vi "main_ctrl.vi"(8 "error in":errorcluster) -> (0 "error out":errorcluster caption="Error")   [LabVIEW 2013]
uses:
  <vilib>/Rock Robotics/WPI/DriverStation/WPI_DriverStationRobotMode2.ctl
  typedefs/Test/test data.ctl
  typedefs/Test/test controls.ctl
  typedefs/fg_typedef.ctl
  typedefs/Vision/vision enable.ctl
  typedefs/State Machine/subStates.ctl
  typedefs/State Machine/singleUseSubstate.ctl
  <vilib>/Rock Robotics/WPI/Solenoid/WPI_SolenoidValue.ctl
  <vilib>/Rock Robotics/WPI/Compressor/WPI_CompressorGetSetRefNum.vi
  <vilib>/Rock Robotics/WPI/RobotDrive/WPI_RobotDriveGetSetRefNum.vi
  <vilib>/Rock Robotics/WPI/RobotDrive/WPI_RobotDriveArcadeDrive_Standard(NoSaturation).vi
  <vilib>/Rock Robotics/WPI/Solenoid/WPI_SolenoidSetEnum.vi
  state machine master/Cancel State Machine - Pickup.vi
  state machine master/Cancel State Machine - Load.vi
  typedefs/Vision/vision data.ctl
panel:
  out "vision errors":errorcluster
  in  "Test\nControls":T1 {"Belts" scale=-1.0..1.0; "Arm" scale=-1.0..1.0; "Drive Train" scale=-1.0..1.0}
  out "Test Data":T2
  out "Robot Mode":T3
  out "Vision mSPI":u32
  out "Vision IPS":dbl
  out "Main IPS":dbl
  out "Main mSPI":u32
  # "Test Input/Output"
  # "MAIN CONTROL"
  # "holds robot control code - dual parallel state machine"
  # "SPI: milliseconds per iteration\nIPS: iterations per second"
  # "Pneumatics"
  # "Home Encoders"
  # "Manual Override"
  # "Joystick Control"
  # "Arm Safeties"
  # "Sensors"
  # "Drive Encoders"
  # "Pneumatics Commands"
  # "Arm Encoder"
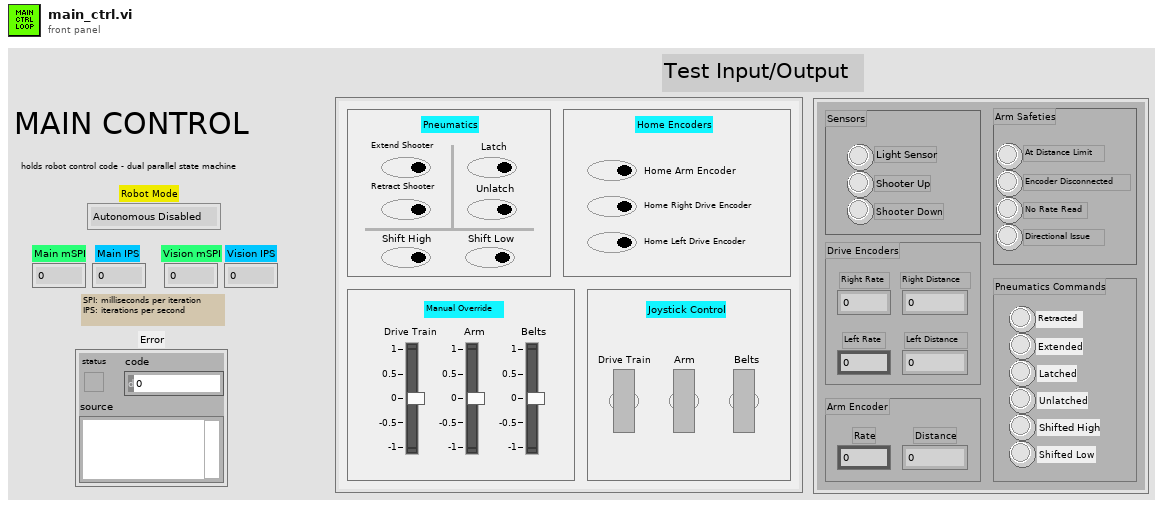
[diagram p1: front panel]
types:
  T1 = typedef "test controls.ctl" = cluster{"Drive Train":dbl, "Arm":dbl, "Belts":dbl, "Drive Train":bool, "Arm":bool, "Belts":bool, "Home Arm Encoder":bool, "Home Right Drive Encoder":bool, "Home Left Drive Encoder":bool, "Extend Shooter":bool, "Retract Shooter":bool, "Latch":bool, "Unlatch":bool, "Shift High":bool, "Shift Low":bool}
  T2 = typedef "test data.ctl" = cluster{"Light Sensor":bool, "Shooter Up":bool, "Shooter Down":bool, "Left Rate":dbl, "Left Distance":dbl, "Right Rate":dbl, "Right Distance":dbl, "Rate":dbl, "Distance":dbl, "At Distance Limit":bool, "Encoder Disconnected":bool, "No Rate Read":bool, "Directional Issue":bool, "Latched":bool, "Unlatched":bool, "Shifted High":bool, "Shifted Low":bool, "Extended":bool, "Retracted":bool}
  T3 = typedef "WPI_DriverStationRobotMode2.ctl" = enum16{"Autonomous Disabled", "Autonomous Enabled", "Teleop Disabled", "Teleop Enabled", "Timeout", "Finish", "Test Disabled", "Test Enabled"}
  T4 = typedef "fg_typedef.ctl" = enum16{"Get", "Set"}
  T5 = typedef "vision data.ctl" = cluster{"x":dbl, "y":dbl, "area":dbl, "width":dbl, "height":dbl, "Hot Goal Present?":bool, "distance":dbl}
  T6 = typedef "vision enable.ctl" = enum16{"Enable", "Disable", "Stop"}
  T7 = typedef "WPI_CameraDevRef.ctl" = cluster{"Camera Address":string, "CameraStatus":errorcluster, "Acquire Image Notifier":refnum<notifier>}
  T8 = typedef "IMAQ Image.ctl" = refnum<image>
  T9 = cluster{"Vision mSPI":u32, "Main mSPI":u32, "Dash mSPI":u32}
  T10 = typedef "WPI_RobotDriveDevRef.ctl" = cluster{"DevStatus":errorcluster, "Motors[]":T11[], "Square Inputs":bool, "Max Output":dbl, "Isochronous":bool}
  T11 = typedef "WPI_MotorControlDeviceRef.ctl" = cluster{"DeviceStatus":errorcluster, "Type":enum16{"PWM", "CAN"}, "PWM":cluster{"Digital Module":T12, "PWM Channel":T13, "DeadBand":T14}, "CAN":cluster{"Device Number":u8, "Control Mode":T15, "Semaphore":T16, "Max Vout":dbl}, "Invert":bool, "TransformRef":T17, "InvTransformRef":T17}
  T12 = typedef "FPGA_TypedefDigitalModule.ctl" = enum16{"Digital Module 1", "Digital Module 2"}
  T13 = typedef "FPGA_DIOPWMChannel.ctl" = enum8{"PWM 1", "PWM 2", "PWM 3", "PWM 4", "PWM 5", "PWM 6", "PWM 7", "PWM 8", "PWM 9", "PWM 10", "Invalid"}
  T14 = typedef "WPI_PWMDeadband.ctl" = cluster{"Name":string, "maxPositivePwm":i32, "minPositivePwm":i32, "centerPwm":i32, "maxNegativePwm":i32, "minNegativePwm":i32, "angularRange":u16}
  T15 = typedef "WPI_CANJaguar_ControlMode.ctl" = enum8{"Percent VBus", "Current", "Speed", "Position", "Voltage"}
  T16 = typedef "Semaphore RefNum" = refnum<k1>
  T17 = typedef "WPI_PWMTransform_ConPane.ctl" = refnum<vi>
  T18 = typedef "WPI_SolenoidDevRef.ctl" = cluster{"DevStatus":errorcluster, "Solenoid Module":T19, "Forward Solenoid Channel":T20, "Reverse Solenoid Channel":T20}
  T19 = typedef "FPGA_TypedefSolenoidModule.ctl" = enum16{"Solenoid Module 1", "Solenoid Module 2"}
  T20 = typedef "WPI_SolenoidChannel.ctl" = enum8{"Solenoid 1", "Solenoid 2", "Solenoid 3", "Solenoid 4", "Solenoid 5", "Solenoid 6", "Solenoid 7", "Solenoid 8", "Invalid"}
  T21 = typedef "WPI_CompressorDevRef.ctl" = cluster{"DevStatus":errorcluster, "DigitalInputDevRef":T22, "RelayDevRef":T24}
  T22 = typedef "WPI_DigitalInputDevRef.ctl" = cluster{"DevStatus":errorcluster, "DIO Channel":T23, "Digital Module":T12}
  T23 = typedef "FPGA_DIOChannel.ctl" = enum8{"DIO 1", "DIO 2", "DIO 3", "DIO 4", "DIO 5", "DIO 6", "DIO 7", "DIO 8", "DIO 9", "DIO 10", "DIO 11", "DIO 12", "DIO 13", "DIO 14", "Invalid"}
  T24 = typedef "WPI_RelayDevRef.ctl" = cluster{"DevStatus":errorcluster, "Relay Channel":T25, "Digital Module":T12, "Relay Direction":T26}
  T25 = typedef "FPGA_DIORelayChannel.ctl" = enum8{"Relay 1", "Relay 2", "Relay 3", "Relay 4", "Relay 5", "Relay 6", "Relay 7", "Relay 8", "Invalid"}
  T26 = typedef "WPI_RelayDirection.ctl" = enum16{"Both directions", "Forward only", "Reverse only"}
  T27 = typedef "WPI_SolenoidValue.ctl" = enum16{"Off", "On", "Forward", "Reverse"}
  T28 = typedef "subStates.ctl" = enum16{"null", "wait", "driver control", "auto", "manual override", "hold position", "rotate", "pickup", "pass", "recover pass", "load", "goto shoot", "shoot high goal", "shoot low goal", "cancel arm", "cancel shooter", "end", "test"}
  T29 = typedef "singleUseSubstate.ctl" = enum16{"null", "wait", "shift high", "shift low", "extend shooter", "retract shooter", "latch", "unlatch", "end"}
  T30 = typedef "WPI_DriverStationDerivedRobotMode.ctl" = enum16{"Init", "Execute", "Stop"}
  T31 = typedef "Loop 2 Datatype.ctl" = cluster{"State":T28, "Waiting Loop":i32, "State to Wait For":i32, "Loop ID":i32, "Exit Value":i32, "Joystick Y":dbl, "Joystick Z":dbl}
  T32 = typedef "Loop 1 Datatype.ctl" = cluster{"State":T28, "Waiting Loop":i32, "State to Wait For":i32, "Loop ID":i32, "Exit Value":i32}
  T33 = typedef "Loop 3 Datatype.ctl" = cluster{"State":T28, "Waiting Loop":i32, "State to Wait For":i32, "Loop ID":i32, "Exit Value":i32, "Joystick Y":dbl, "Tune Setpoint":cluster{"Increment":bool, "Decrement":bool}}
  T34 = typedef "Loop 0 Datatype.ctl" = cluster{"State":T28, "Waiting Loop":i32, "State to Wait For":i32, "Loop ID":i32, "Exit Value":i32, "X Axis":dbl, "Y Axis":dbl, "Z Axis":dbl}
  T35 = typedef "dashboard safety status data.ctl" = cluster{"At Distance Limit":bool, "No Rate Read":bool, "Encoder Disconnected":bool, "Encoder Directional Issue":bool}
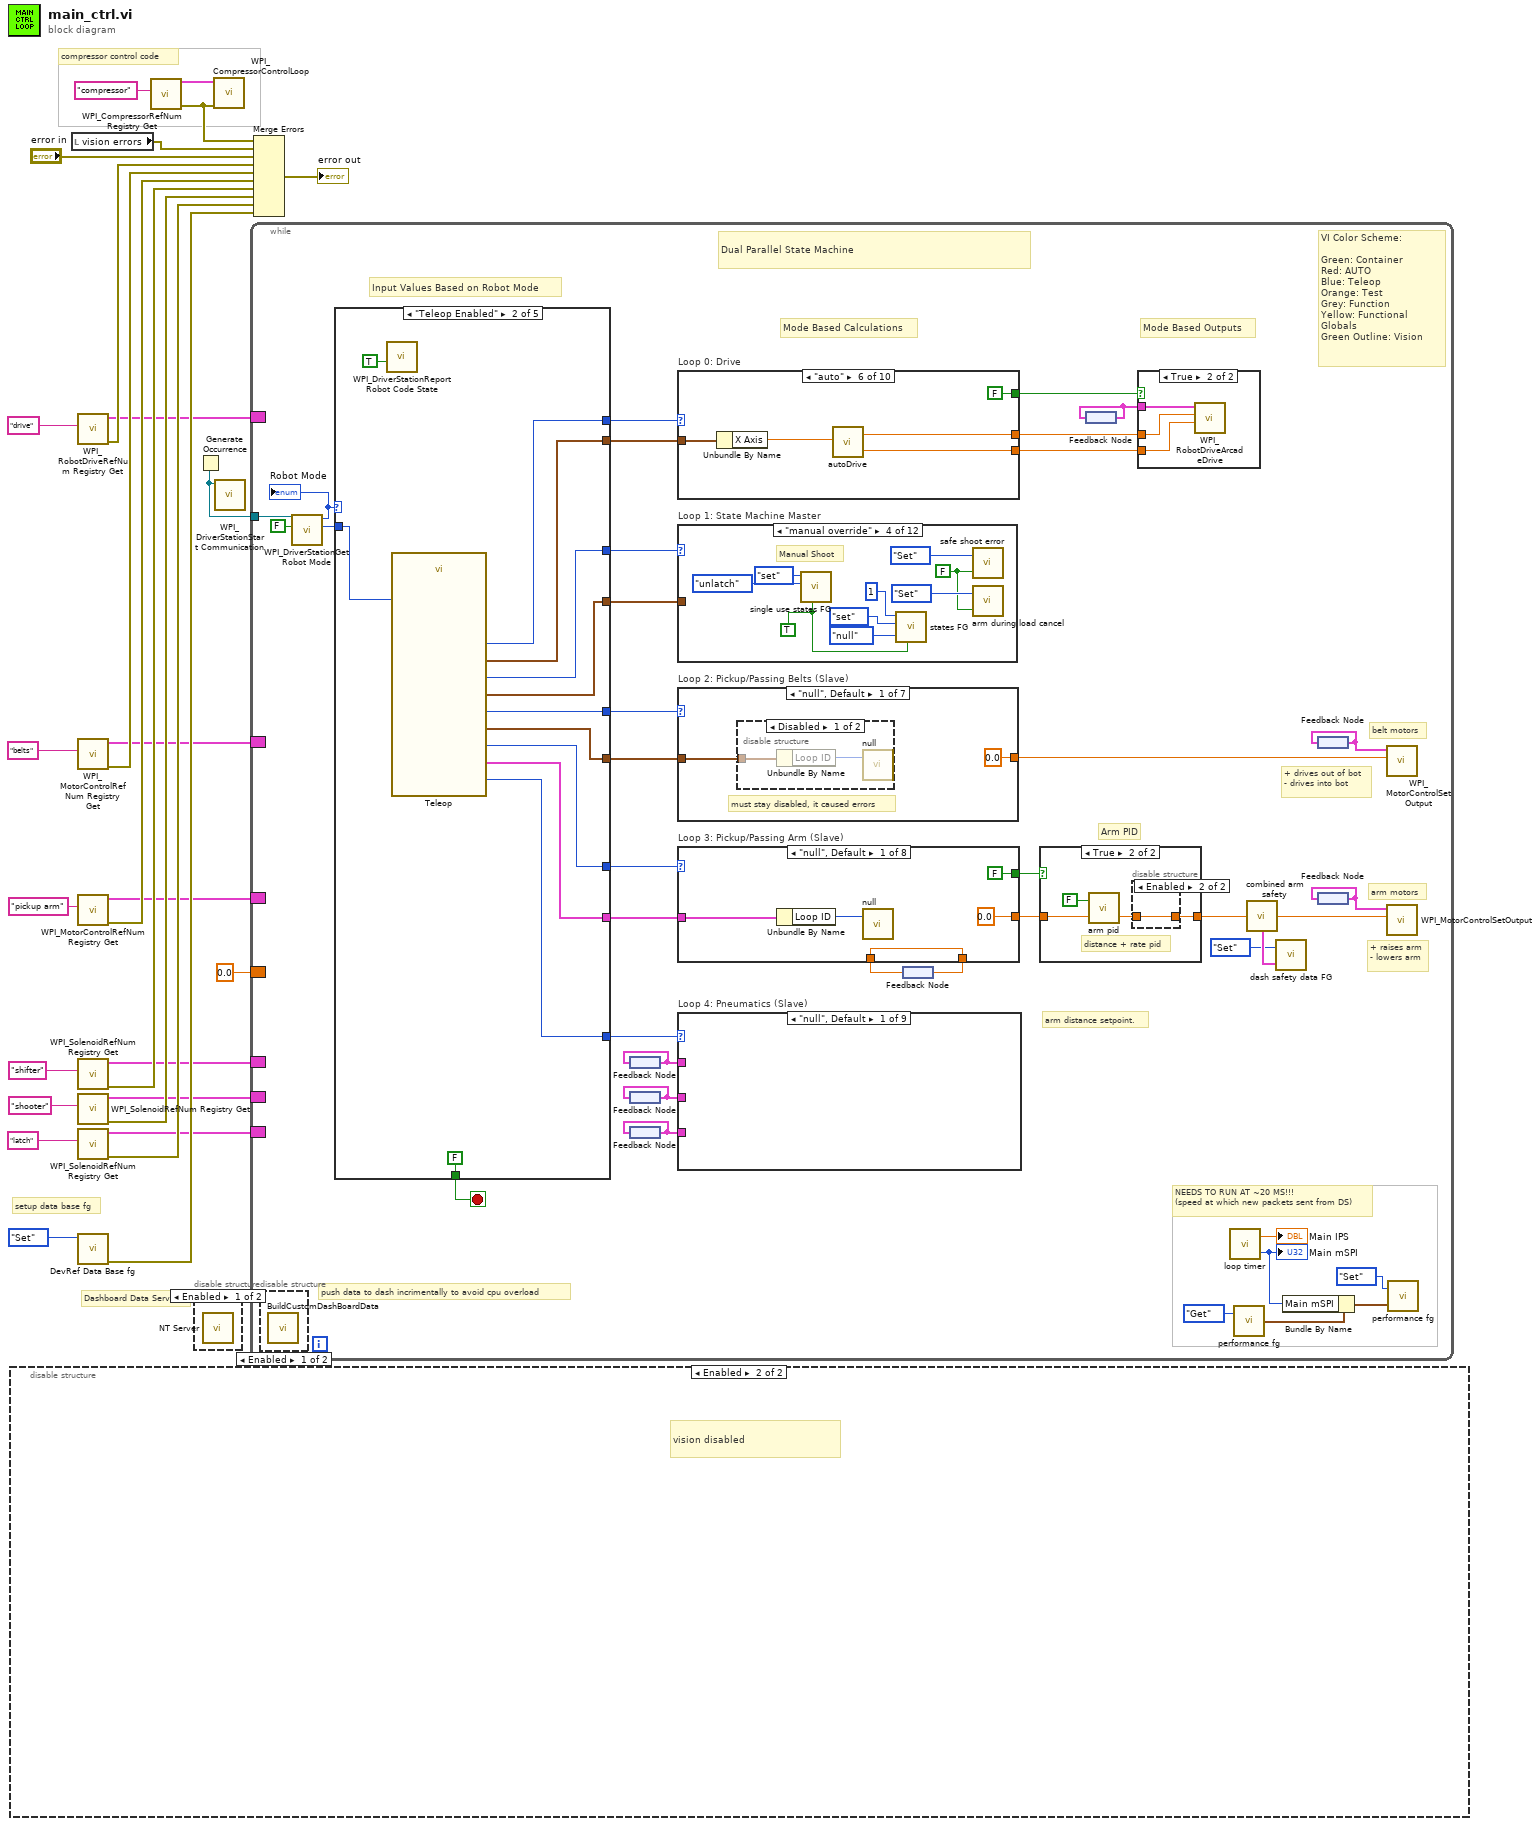
[diagram p0: block diagram]
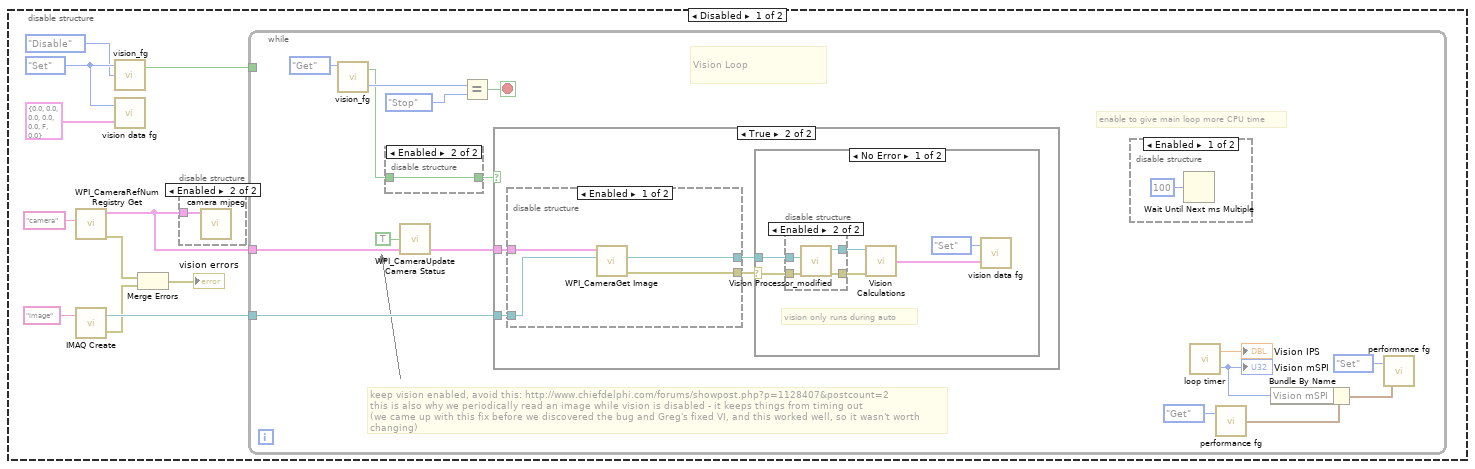
[diagram p3: hidden frame]
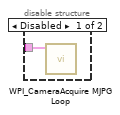
[diagram p4: hidden frame]
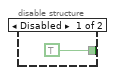
[diagram p5: hidden frame]
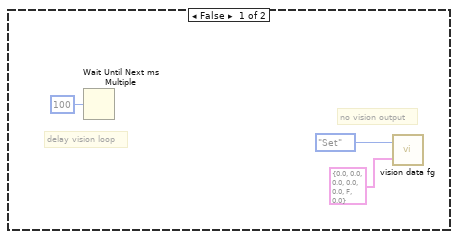
[diagram p7: hidden frame]
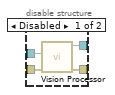
[diagram p8: hidden frame]
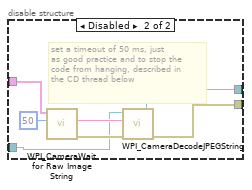
[diagram p10: hidden frame]
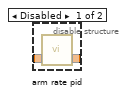
[diagram p12: hidden frame]
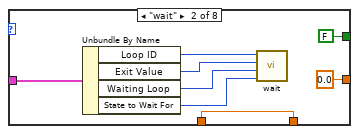
[diagram p13: hidden frame]
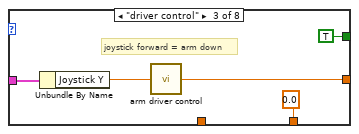
[diagram p14: hidden frame]
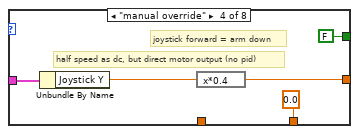
[diagram p15: hidden frame]
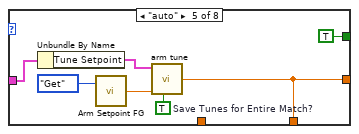
[diagram p16: hidden frame]
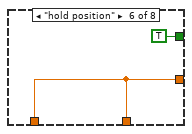
[diagram p17: hidden frame]
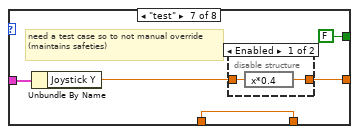
[diagram p18: hidden frame]
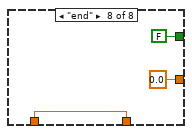
[diagram p20: hidden frame]
diagram:
  # "compressor control code"
  # "Dashboard Data Server"
  # "setup data base fg"
  n1 = disable-structure shown="Enabled" {
    frame Disabled {
      w37 = fg_typedef."Set" ("Enum")
      n2 = call <vilib>:"WPI_CameraRefNum Registry Get.vi"("refnum name"="camera") -> ("error out"=w30:errorcluster, "CameraDevRef"=w34:T7)  [unwired: 9 in]
      n3 = call "IMAQ Create"("Image Name"="image") -> ("New Image"=w39:T8, "error out"=w31:errorcluster)  [unwired: 4 in]
      n4 = call "vision_fg.vi"("Action"=vision_enable."Disable", "Menu"=w37) -> ("Enabled?"=w38:bool)  [unwired: 1 in, 1 out]
      n5 = call "vision data fg.vi"("Input"=T5 {"x"=0.0, "y"=0.0, "area"=0.0, "width"=0.0, "height"=0.0, "Hot Goal Present?"=FALSE, "distance"=0.0} ("Cluster"), "Menu"=w37) -> ()  [unwired: 1 out]
      n6 = Merge Errors(w30, w31) -> (→"vision errors":errorcluster)
      n7 = disable-structure shown="Enabled" {
        disable-tunnel: w34 -> [w40 w41]
        frame Disabled {
          n8 = call <vilib>:"WPI_CameraAcquire MJPG Loop.vi"("CameraDevRef"=w40) -> ()  [unwired: 11 in]
        }
        frame Enabled {
          n9 = call "camera mjpeg.vi"("CameraDevRef"=w41) -> ()  [unwired: 11 in]
        }
      }
      n10 = while {
        tunnel: w39 -> [w56]
        tunnel: w34 -> [w55]
        tunnel: w38 -> [_]
        stop <- w57 stop-if-true
        # "keep vision enabled, avoid this: http://www.chiefdelphi.com/forums/showpost.php?p=1128407&postcount=2\nthis is also why we periodically read an image while vision is disabled - it keeps things from timing out\n(we came up with this fix before we discovered the bug and Greg's fixed VI, and this worked well, so it wasn't worth changing)"
        # "enable to give main loop more CPU time"
        # "Vision Loop"
        n11 = call "vision_fg.vi"("Menu"=fg_typedef."Get" ("Enum")) -> ("State Out"=w51:T6, "Enabled?"=w42:bool)  [unwired: 2 in]
        n12 = disable-structure shown="Enabled" {
          disable-tunnel: [TRUE w59] -> w43
          disable-tunnel: w42 -> [_ w59]
          frame Disabled {
          }
          frame Enabled {
          }
        }
        n13 = call <vilib>:"WPI_CameraUpdate Camera Status.vi"("CameraDevRef In"=w55, "Enable Vision"=TRUE) -> ("CameraDevRef Out"=w54:T7)  [unwired: 3 in]
        n14 = Equal?(x=w51, y=vision_enable."Stop") -> (x = y?=w57:bool)
        n15 = case shown="True" w43 {
          tunnel: w56 -> [_ w67]
          tunnel: w54 -> [_ w66]
          frame False {
            # "no vision output"
            # "delay vision loop"
            n16 = Wait Until Next ms Multiple(millisecond multiple=u32 100) -> ()  [unwired: 1 out]
            n17 = call "vision data fg.vi"("Input"=T5 {"x"=0.0, "y"=0.0, "area"=0.0, "width"=0.0, "height"=0.0, "Hot Goal Present?"=FALSE, "distance"=0.0} ("Cluster"), "Menu"=fg_typedef."Set" ("Enum")) -> ()  [unwired: 1 out]
          }
          frame True {
            n18 = disable-structure shown="Enabled" {
              disable-tunnel: w67 -> [w84 w88]
              disable-tunnel: w66 -> [w85 w90]
              disable-tunnel: [w83 w87] -> w65
              disable-tunnel: [w82 w86] -> w64
              frame Enabled {
                n19 = call <vilib>:"WPI_CameraGet Image.vi"("Image"=w84, "CameraDevRef"=w85) -> ("error out"=w82:errorcluster, "Image Out"=w83:T8)  [unwired: 7 in, 1 out]
              }
              frame Disabled {
                # "set a timeout of 50 ms, just\nas good practice and to stop the \ncode from hanging, described in \nthe CD thread below"
                n20 = call <vilib>:"WPI_CameraWait for Raw Image String.vi"("Timeout in ms (-1)"=50, "CameraDevRef"=w90) -> ("error out"=w92:errorcluster, "String"=w91:string)  [unwired: 3 in, 5 out]
                n21 = call <vilib>:"WPI_CameraDecodeJPEGString.vi"("error in"=w92, "Compressed Image"=w91, "Image In"=w88) -> ("error out"=w86:errorcluster, "Image Out"=w87:T8)  [unwired: 3 out]
              }
            }
            n22 = case shown="No Error" w64 {
              selector: w64 -> [w72 _]
              tunnel: w65 -> [w71 _]
              frame No Error {
                # "vision only runs during auto"
                n23 = disable-structure shown="Enabled" {
                  disable-tunnel: w72 -> [w77 w80]
                  disable-tunnel: w71 -> [w76 w81]
                  disable-tunnel: [w75 w78] -> w70
                  disable-tunnel: [w74 w79] -> w69
                  frame Disabled {
                    n24 = call "Vision Processor.vi"("error in"=w77, "Image In"=w76) -> ("error out"=w74:errorcluster, "Image Out"=w75:T8)  [unwired: 5 in]
                  }
                  frame Enabled {
                    n25 = call "Vision Processor_modified.vi"("error in"=w80, "Image In"=w81) -> ("error out"=w79:errorcluster, "Image Out"=w78:T8)  [unwired: 5 in]
                  }
                }
                n26 = call "Vision Calculations.vi"("Image In"=w70, "error in"=w69) -> ("Vision Data"=w68:T5)  [unwired: 3 in]
                n27 = call "vision data fg.vi"("Input"=w68, "Menu"=fg_typedef."Set" ("Enum")) -> ()  [unwired: 1 out]
              }
              frame Error {
              }
            }
          }
        }
        n28 = disable-structure shown="Enabled" {
          frame Enabled {
            n29 = Wait Until Next ms Multiple(millisecond multiple=u32 100) -> ()  [unwired: 1 out]
          }
          frame Disabled {
          }
        }
        n30 = call "loop timer.vi"() -> ("IPS"=→"Vision IPS":dbl, "SPI"=w49:u32)  [unwired: 1 in]
        "Vision mSPI" <- w49
        n31 = call "performance fg.vi"("Menu"=fg_typedef."Get") -> ("Output"=w47:T9)  [unwired: 1 in]
        n32 = Bundle By Name(cluster=w47, "Vision mSPI"=w49) -> (w46:T9)
        n33 = call "performance fg.vi"("Input"=w46, "Menu"=fg_typedef."Set") -> ()  [unwired: 1 out]
      }
    }
    frame Enabled {
      # "vision disabled"
    }
  }
  n34 = local read "vision errors"() -> (w1:errorcluster)
  n35 = call <vilib>:"WPI_RobotDriveRefNum Registry Get.vi"("refnum name"="drive") -> ("error out"=w27:errorcluster, "RobotDriveDevRef"=w3:T10)  [unwired: 9 in]
  n36 = call <vilib>:"WPI_MotorControlRefNum Registry Get.vi"("refnum name"="belts") -> ("error out"=w26:errorcluster, "MotorControlDevRef"=w7:T11)  [unwired: 9 in]
  n37 = call <vilib>:"WPI_MotorControlRefNum Registry Get.vi"("refnum name"="pickup arm") -> ("error out"=w25:errorcluster, "MotorControlDevRef"=w10:T11)  [unwired: 9 in]
  n38 = call <vilib>:"WPI_SolenoidRefNum Registry Get.vi"("refnum name"="shifter") -> ("error out"=w24:errorcluster, "SolenoidDevRef"=w17:T18)  [unwired: 9 in]
  n39 = call <vilib>:"WPI_SolenoidRefNum Registry Get.vi"("refnum name"="shooter") -> ("error out"=w23:errorcluster, "SolenoidDevRef"=w5:T18)  [unwired: 9 in]
  n40 = call <vilib>:"WPI_SolenoidRefNum Registry Get.vi"("refnum name"="latch") -> ("error out"=w22:errorcluster, "SolenoidDevRef"=w6:T18)  [unwired: 9 in]
  n41 = call "DevRef Data Base fg.vi"("Menu"=fg_typedef."Set") -> ("error out"=w28:errorcluster)  [unwired: 3 in, 5 out]
  n42 = call <vilib>:"WPI_CompressorRefNum Registry Get.vi"("refnum name"="compressor") -> ("error out"=w2:errorcluster, "CompressorDevRef"=w18:T21)  [unwired: 9 in]
  n43 = disable-structure shown="Enabled" {
    frame Enabled {
      n44 = call <vilib>:"NT Server.vi"() -> ()  [unwired: 12 in]
    }
    frame Disabled {
    }
  }
  n45 = Generate Occurrence() -> (w15:refnum<k4>)
  n46 = call <vilib>:"WPI_CompressorControlLoop.vi"("error in (no error)"=w2, "CompressorDevRef"=w18) -> ()  [unwired: 10 in]
  n47 = call <vilib>:"WPI_DriverStationStart Communication.vi"("occurrence"=w15) -> ()  [unwired: 11 in]
  n48 = while {
    tunnel: w15 -> [w110]
    border: w3 -> [_]
    border: w17 -> [_]
    border: w6 -> [_]
    border: w5 -> [_]
    border: w7 -> [_]
    border: w10 -> [_]
    border: 0.0 ("setpoint") -> [_]
    stop <- w127 stop-if-true
    # "Arm PID"
    # "Mode Based Outputs"
    # "arm motors"
    # "arm distance setpoint."
    # "push data to dash incrimentally to avoid cpu overload"
    # "+ raises arm\n- lowers arm"
    # "+ drives out of bot\n- drives into bot"
    # "belt motors"
    # "VI Color Scheme:\n\nGreen: Container\nRed: AUTO\nBlue: Teleop\nOrange: Test \nGrey: Function\nYellow: Functional Globals\nGreen Outline: Vision"
    # "Input Values Based on Robot Mode"
    # "Mode Based Calculations"
    # "NEEDS TO RUN AT ~20 MS!!!\n(speed at which new packets sent from DS)"
    # "Dual Parallel State Machine"
    n49 = disable-structure shown="Enabled" {
      frame Enabled {
        n50 = call "BuildCustomDashBoardData.vi"() -> ()  [unwired: 12 in]
      }
      frame Disabled {
      }
    }
    n51 = call <vilib>:"WPI_DriverStationGet Robot Mode.vi"("Finish"=FALSE, "DS Occurrence"=w110) -> ("Call Context"=w109:T30, "Robot Mode"=w108:T3)  [unwired: 8 out]
    "Robot Mode" <- w108
    n52 = case shown="\"Teleop Enabled\"" w108 {
      tunnel: [w316 w331 w340 w348 w354] -> w112
      tunnel: w109 -> [w309 w327 w343 _ _]
      tunnel: [w314 w330 w342 w348 w354] -> w129
      tunnel: [w310 w328 w334 singleUseSubstate."null" ("SubState 5") singleUseSubstate."end" ("SubState 5")] -> w128
      tunnel: [FALSE FALSE FALSE FALSE TRUE] -> w127
      tunnel: [w318 w326 w338 w348 w354] -> w102
      tunnel: [w317 w325 w339 _ _] -> w121
      tunnel: [w315 w324 w341 _ _] -> w120
      tunnel: [w313 w323 w337 _ _] -> w119
      tunnel: [w311 w322 w335 _ _] -> w117
      tunnel: [w312 w321 w336 w348 w354] -> w101
      frame "Autonomous Enabled" {
        n53 = call <vilib>:"WPI_DriverStationReport Robot Code State.vi"("Autonomous"=TRUE) -> ()  [unwired: 10 in, 1 out]
        n54 = call "Autonomous.vi"("Call Context"=w309) -> ("SubState 2"=w314:T28, "Loop 2 Data"=w313:T31, "SubState 1"=w316:T28, "Loop 1 Data"=w315:T32, "Loop 3 Data"=w311:T33, "SubState 0"=w318:T28, "SubState 3"=w312:T28, "Loop 0 Data"=w317:T34, "SubState 4"=w310:T29)  [unwired: 2 in]
      }
      frame "Teleop Enabled" {
        n55 = call <vilib>:"WPI_DriverStationReport Robot Code State.vi"("TeleOp"=TRUE) -> ()  [unwired: 10 in, 1 out]
        n56 = call "Teleop.vi"("Call Context"=w327) -> ("SubState 3"=w321:T28, "SubState 4"=w328:T29, "Loop 3 Data"=w322:T33, "SubState 0"=w326:T28, "Loop 1 Data"=w324:T32, "Loop 0 Data"=w325:T34, "SubState 1"=w331:T28, "Loop 2 Data"=w323:T31, "SubState 2"=w330:T28)  [unwired: 10 in]
      }
      frame "Test Enabled" {
        n57 = call <vilib>:"WPI_DriverStationReport Robot Code State.vi"("Test"=TRUE) -> ()  [unwired: 10 in, 1 out]
        n58 = call "Test.vi"("Test Controls"="Test\nControls", "Call Context"=w343) -> ("Loop 2 Data"=w337:T31, "SubState 2"=w342:T28, "Loop 1 Data"=w341:T32, "SubState 1"=w340:T28, "SubState 3"=w336:T28, "Loop 0 Data"=w339:T34, "Loop 3 Data"=w335:T33, "SubState 0"=w338:T28, "SubState 4"=w334:T29, "Test Data"=→"Test Data":T2)
      }
      frame "Autonomous Disabled", "Teleop Disabled", "Timeout", "Test Disabled" {
        w348 = subStates."null" ("SubState 0")
        # "set all loops to null"
        # "make sure to disable vision\nwe don't need it here"
        # "robot disabled, timeout"
        n59 = call <vilib>:"WPI_DriverStationReport Robot Code State.vi"("Disabled"=TRUE) -> ()  [unwired: 10 in, 1 out]
        n60 = call "vision_fg.vi"("Action"=vision_enable."Disable", "Menu"=fg_typedef."Set") -> ()  [unwired: 1 in, 2 out]
      }
      frame "Finish" {
        w354 = subStates."end" ("Loop State")
        # "Stop All Loops"
        # "stop the while loop"
        # "stop DS comms"
        # "stop vision loop"
        n61 = call <vilib>:"WPI_DriverStationStop Communication.vi"("StopCommunication"=TRUE) -> ()  [unwired: 10 in, 1 out]
        n62 = call "vision_fg.vi"("Action"=vision_enable."Stop", "Menu"=fg_typedef."Set") -> ()  [unwired: 1 in, 2 out]
      }
    }
    n63 = feedback #1() -> (w118:T18)
    n64 = feedback-in #1(w118) -> ()
    n65 = feedback #2() -> (w104:T18)
    n66 = feedback-in #2(w104) -> ()
    n67 = feedback #3() -> (w103:T18)
    n68 = feedback-in #3(w103) -> ()
    n69 = case "Loop 0: Drive" shown="\"auto\"" w102 {
      tunnel: w121 -> [w216 w221 w231 w243 w251 w254 w260 _ w273 _]
      tunnel: [w215 w220 w230 w240 w248 w256 w262 w264 0.0 ("X Axis") w275] -> w115
      tunnel: [w215 w220 w229 w239 w247 w255 w261 w263 w272 w275] -> w114
      tunnel: [FALSE FALSE TRUE FALSE FALSE FALSE FALSE FALSE TRUE FALSE] -> w116
      frame "null", Default {
        w215 = 0.0 ("X Axis")
        n70 = disable-structure shown="Enabled" {
          disable-tunnel: w216 -> [w218 _]
          frame Disabled {
            n71 = Unbundle By Name(w218) -> ("Loop ID"=w217:i32)
            n72 = call "null.vi"("This Loop ID"=w217) -> ()  [unwired: 2 in]
          }
          frame Enabled {
          }
        }
      }
      frame "wait" {
        w220 = 0.0 ("X Axis")
        n73 = Unbundle By Name(w221) -> ("Loop ID"=w225:i32, "Exit Value"=w224:i32, "Waiting Loop"=w223:i32, "State to Wait For"=w222:i32)
        n74 = call "wait.vi"("State to wait for"=w222, "Waiting Loop ID"=w223, "time (ms)"=w224, "Current Loop ID"=w225) -> ()  [unwired: 1 out]
      }
      frame "driver control" {
        n75 = Unbundle By Name(w231) -> ("X Axis"=w227:dbl, "Y Axis"=w228:dbl)
        n76 = disable-structure shown="Enabled" {
          disable-tunnel: w227 -> [w235 w237]
          disable-tunnel: w228 -> [w234 w236]
          disable-tunnel: [w233 w237] -> w230
          disable-tunnel: [w232 w236] -> w229
          frame Disabled {
            n77 = call "calc arcade drive pwm.vi"("Y axis value"=w234, "X axis value"=w235) -> ("Right Speed"=w232:dbl, "Left Speed"=w233:dbl)  [unwired: 1 in, 1 out]
          }
          frame Enabled {
          }
        }
      }
      frame "manual override" {
        n78 = Unbundle By Name(w243) -> ("X Axis"=w242:dbl, "Y Axis"=w241:dbl)
        n79 = expression code="x/2"(w242) -> (w240:dbl)
        n80 = expression code="x/2"(w241) -> (w239:dbl)
      }
      frame "hold position" {
        n81 = Unbundle By Name(w251) -> ("X Axis"=w250:dbl, "Y Axis"=w249:dbl)
        n82 = call "closed drive.vi"("Acrade Drive?"=TRUE, "Y axis value (Left)"=w249, "X axis value (Right)"=w250, "Threshold (.4)"=0.4) -> ("right"=w247:dbl, "left"=w248:dbl)
      }
      frame "auto" {
        n83 = Unbundle By Name(w254) -> ("X Axis"=w252:dbl)
        n84 = call "autoDrive.vi"("Distance"=w252) -> ("right speed"=w255:dbl, "left speed"=w256:dbl)  [unwired: 2 in, 1 out]
      }
      frame "rotate" {
        n85 = Unbundle By Name(w260) -> ("X Axis"=w259:dbl, "Y Axis"=w258:dbl)
        n86 = call "rotate.vi"("Rate"=w258, "Angle"=w259) -> ("right speed"=w261:dbl, "left speed"=w262:dbl)  [unwired: 1 in, 1 out]
      }
      frame "goto shoot" {
        n87 = disable-structure shown="Enabled" {
          disable-tunnel: [w267 _] -> w264
          disable-tunnel: [w266 _] -> w263
          frame Disabled {
            # "consider implimenting closed hold with drive"
            n88 = call "vision data fg.vi"("Menu"=fg_typedef."Get") -> ("Output"=w268:T5)  [unwired: 1 in]
            n89 = call "goto location.vi"("Image Data"=w268) -> ("left speed"=w267:dbl, "right speed"=w266:dbl)
          }
          frame Enabled {
            # "not going to do this"
          }
        }
      }
      frame "test" {
        n90 = Unbundle By Name(w273) -> ("Y Axis"=w272:dbl)
      }
      frame "end" {
        w275 = 0.0 ("X Axis")
      }
    }
    n91 = case "Loop 1: State Machine Master" shown="\"manual override\"" w112 {
      tunnel: w120 -> [w293 w294 _ _ _ _ _ _ _ _ _ _]
      frame "null", Default {
        n92 = Unbundle By Name(w293) -> ("Loop ID"=w292:i32)
        n93 = call "null.vi"("This Loop ID"=w292) -> ()  [unwired: 2 in]
      }
      frame "wait" {
        n94 = Unbundle By Name(w294) -> ("Loop ID"=w298:i32, "Exit Value"=w297:i32, "Waiting Loop"=w296:i32, "State to Wait For"=w295:i32)
        n95 = call "wait.vi"("State to wait for"=w295, "Waiting Loop ID"=w296, "time (ms)"=w297, "Current Loop ID"=w298) -> ()  [unwired: 1 out]
      }
      frame "auto" {
        # "A State Machine for Auto"
        n96 = call "Auto State Machine.vi"() -> ()  [unwired: 12 in]
      }
      frame "manual override" {
        w304 = FALSE ("Can Shoot Safely?")
        w299 = TRUE ("exit in")
        # "Manual Shoot"
        n97 = call "single use states FG.vi"("exit in"=w299, "substate"=singleUseSubstate."unlatch", "menu (get)"=enum16{"set", "get"}."set") -> ()  [unwired: 5 in, 4 out]
        n98 = call "states FG.vi"("exit in"=w299, "subState in"=subStates."null", "menu (get)"=enum16{"set", "get"}."set", "Loop ID"=1) -> ()  [unwired: 4 in, 4 out]
        n99 = call "safe shoot error.vi"("Can Shoot Safely?"=w304, "Menu"=fg_typedef."Set") -> ()  [unwired: 1 out]
        n100 = call "arm during load cancel.vi"("Arm Canceled During Load?"=w304, "Mode"=enum16{"Get", "Set", "Teleop Set"}."Set") -> ()  [unwired: 1 out]
      }
      frame "pickup" {
        # "A State Machine for Pickup"
        n101 = call "Pickup State Machine.vi"() -> ()  [unwired: 12 in]
      }
      frame "pass" {
        # "A State Machine for Passing"
        n102 = call "Pass State Machine.vi"() -> ()  [unwired: 12 in]
      }
      frame "recover pass" {
        # "If a pass fails i.e. ball gets stuck, let the drivers fix it"
        # "A State Machine for Recovering a Pass"
        n103 = call "Pass Recovery State Machine.vi"() -> ()  [unwired: 12 in]
      }
      frame "load" {
        # "ball can now (after this) be high or low goal shot"
        # "A State Machine for Loading"
        n104 = call "Load State Machine.vi"() -> ()  [unwired: 12 in]
      }
      frame "shoot high goal" {
        # "A State Machine for High Goal Shooting"
        n105 = call "Shoot High Goal State Machine.vi"() -> ()  [unwired: 12 in]
      }
      frame "shoot low goal" {
        # "A State Machine for Low Goal Shooting"
        n106 = call "Shoot Low Goal State Machine.vi"() -> ()  [unwired: 12 in]
      }
      frame "cancel arm" {
        # "A State Machine for Canceling Pickup"
        n107 = call-poly "Cancel State Machine - Polymorphic.vi"() -> ()  [unwired: 1 in]
      }
      frame "cancel shooter" {
        # "A State Machine for Canceling Load"
        n108 = call-poly "Cancel State Machine - Polymorphic.vi"() -> ()  [unwired: 1 in]
      }
    }
    n109 = case "Loop 2: Pickup/Passing Belts (Slave)" shown="\"null\", Default" w129 {
      tunnel: w119 -> [w183 w187 w194 w197 w204 w206 _]
      tunnel: [0.0 ("output") 0.0 ("output") w192 w195 w201 w205 0.0 ("Joystick Y")] -> w105
      frame "null", Default {
        # "must stay disabled, it caused errors"
        n110 = disable-structure shown="Disabled" {
          disable-tunnel: w183 -> [w185 _]
          frame Disabled {
            n111 = Unbundle By Name(w185) -> ("Loop ID"=w184:i32)
            n112 = call "null.vi"("This Loop ID"=w184) -> ()  [unwired: 2 in]
          }
          frame Enabled {
          }
        }
      }
      frame "wait" {
        n113 = Unbundle By Name(w187) -> ("Loop ID"=w191:i32, "Exit Value"=w190:i32, "Waiting Loop"=w189:i32, "State to Wait For"=w188:i32)
        n114 = call "wait.vi"("State to wait for"=w188, "Waiting Loop ID"=w189, "time (ms)"=w190, "Current Loop ID"=w191) -> ()  [unwired: 1 out]
      }
      frame "driver control" {
        # "which joystick? should be specified in name."
        # "joystick forward = out of bot"
        n115 = Unbundle By Name(w194) -> ("Joystick Y"=w193:dbl)
        n116 = Negate(x=w193) -> (-x=w192:dbl)
      }
      frame "manual override" {
        # "essentially driver control, but 1/2 speed?"
        # "joystick forward = out of bot"
        n117 = Unbundle By Name(w197) -> ("Joystick Y"=w196:dbl)
        n118 = expression code="-x/2"(w196) -> (w195:dbl)
      }
      frame "auto" {
        # "get speed to go as set by master and tune"
        n119 = Unbundle By Name(w204) -> ("Joystick Z"=w202:dbl)
        n120 = call "Joystick tuner.vi"("Joystick Z"=w202, "Loop ID"=2) -> ("Output"=w200:dbl)  [unwired: 7 in]
        n121 = call "Belt Speed FG.vi"("Menu"=fg_typedef."Get") -> ("Speed Out"=w199:dbl)  [unwired: 1 in]
        n122 = Multiply(x=w200, y=w199) -> (x*y=w201:dbl)
      }
      frame "test" {
        n123 = Unbundle By Name(w206) -> ("Joystick Y"=w205:dbl)
      }
      frame "end" {
      }
    }
    n124 = case "Loop 4: Pneumatics (Slave)" shown="\"null\", Default" w128 {
      tunnel: w118 -> [_ _ w277 w278 _ _ _ _ _]
      tunnel: w104 -> [_ _ _ _ w280 w282 _ _ w290]
      tunnel: w103 -> [_ _ _ _ _ _ w284 w286 w288]
      frame "null", Default {
      }
      frame "wait" {
      }
      frame "shift high" {
        n125 = call-poly <vilib>:"WPI_SolenoidSet.vi"("Value"=WPI_SolenoidValue."Forward", "SolenoidDevRef"=w277) -> ()  [unwired: 8 in, 2 out]
      }
      frame "shift low" {
        n126 = call-poly <vilib>:"WPI_SolenoidSet.vi"("Value"=WPI_SolenoidValue."Reverse", "SolenoidDevRef"=w278) -> ()  [unwired: 8 in, 2 out]
      }
      frame "extend shooter" {
        n127 = call-poly <vilib>:"WPI_SolenoidSet.vi"("Value"=WPI_SolenoidValue."Forward", "SolenoidDevRef"=w280) -> ()  [unwired: 8 in, 2 out]
      }
      frame "retract shooter" {
        n128 = call-poly <vilib>:"WPI_SolenoidSet.vi"("Value"=WPI_SolenoidValue."Reverse", "SolenoidDevRef"=w282) -> ()  [unwired: 8 in, 2 out]
      }
      frame "latch" {
        # "When the latch piston\nis reversed, the latch\nis closed. When the\nlatch piston is\nextended, the latch is\nopen."
        n129 = call-poly <vilib>:"WPI_SolenoidSet.vi"("Value"=WPI_SolenoidValue."Reverse", "SolenoidDevRef"=w284) -> ()  [unwired: 8 in, 2 out]
      }
      frame "unlatch" {
        # "When the latch piston\nis reversed, the latch\nis closed. When the\nlatch piston is\nextended, the latch is\nopen."
        n130 = call-poly <vilib>:"WPI_SolenoidSet.vi"("Value"=WPI_SolenoidValue."Forward", "SolenoidDevRef"=w286) -> ()  [unwired: 8 in, 2 out]
      }
      frame "end" {
        # "retract shooter and unlatch"
        n131 = call-poly <vilib>:"WPI_SolenoidSet.vi"("Value"=WPI_SolenoidValue."Reverse", "SolenoidDevRef"=w290) -> ()  [unwired: 8 in, 2 out]
        n132 = call-poly <vilib>:"WPI_SolenoidSet.vi"("Value"=WPI_SolenoidValue."Forward", "SolenoidDevRef"=w288) -> ()  [unwired: 8 in, 2 out]
      }
    }
    n133 = feedback #4() -> (w96:dbl)
    n134 = case "Loop 3: Pickup/Passing Arm (Slave)" shown="\"null\", Default" w101 {
      tunnel: w117 -> [w143 w147 w155 w161 w168 _ w175 _]
      tunnel: [FALSE FALSE TRUE FALSE TRUE TRUE FALSE FALSE] -> w99
      tunnel: [0.0 ("output") 0.0 ("output") w154 w159 w162 w169 w171 0.0 ("Joystick Y")] -> w98
      tunnel: [w140 w144 0.0 ("setpoint") 0.0 ("setpoint") w162 w169 w172 w179] -> w97
      tunnel: w96 -> [w140 w144 _ _ _ w169 w172 w179]
      frame "null", Default {
        n135 = Unbundle By Name(w143) -> ("Loop ID"=w139:i32)
        n136 = call "null.vi"("This Loop ID"=w139) -> ()  [unwired: 2 in]
      }
      frame "wait" {
        n137 = Unbundle By Name(w147) -> ("Loop ID"=w151:i32, "Exit Value"=w150:i32, "Waiting Loop"=w149:i32, "State to Wait For"=w148:i32)
        n138 = call "wait.vi"("State to wait for"=w148, "Waiting Loop ID"=w149, "time (ms)"=w150, "Current Loop ID"=w151) -> ()  [unwired: 1 out]
      }
      frame "driver control" {
        # "joystick forward = arm down"
        n139 = Unbundle By Name(w155) -> ("Joystick Y"=w153:dbl)
        n140 = call "arm driver control.vi"("Joystick Y"=w153) -> ("Setpoint"=w154:dbl)
      }
      frame "manual override" {
        # "half speed as dc, but direct motor output (no pid)"
        # "joystick forward = arm down"
        n141 = Unbundle By Name(w161) -> ("Joystick Y"=w160:dbl)
        n142 = expression code="x*0.4"(w160) -> (w159:dbl)
      }
      frame "auto" {
        w163 = TRUE  # Save Tunes for Entire Match?
        n143 = Unbundle By Name(w168) -> ("Tune Setpoint"=w165:cluster{"Increment":bool, "Decrement":bool})
        n144 = call "Arm Setpoint FG.vi"("Menu"=fg_typedef."Get") -> ("Setpoint Out"=w164:dbl)  [unwired: 1 in]
        n145 = call "arm tune.vi"("Tune Data"=w165, "Setpoint"=w164, "Save Tunes for Entire Match?"=w163) -> ("Tuned Setpoint"=w162:dbl)  [unwired: 4 in]
      }
      frame "hold position" {
      }
      frame "test" {
        # "need a test case so to not manual override\n(maintains safeties)"
        n146 = Unbundle By Name(w175) -> ("Joystick Y"=w174:dbl)
        n147 = disable-structure shown="Enabled" {
          disable-tunnel: w174 -> [w177 w178]
          disable-tunnel: [w176 w178] -> w171
          frame Enabled {
            n148 = expression code="x*0.4"(w177) -> (w176:dbl)
          }
          frame Disabled {
          }
        }
      }
      frame "end" {
      }
    }
    n149 = feedback-in #4(w97) -> ()
    n150 = case shown="True" w99 {
      tunnel: w98 -> [w131 w134]
      tunnel: [w131 w132] -> w93
      frame False {
        # "open loop"
      }
      frame True {
        # "distance + rate pid"
        n151 = call "arm pid.vi"("Setpoint"=w134, "Autotune?"=FALSE) -> ("Output"=w133:dbl)  [unwired: 1 in]
        n152 = disable-structure shown="Enabled" {
          disable-tunnel: w133 -> [w137 w138]
          disable-tunnel: [w136 w138] -> w132
          frame Disabled {
            n153 = call "arm rate pid.vi"("Rate In"=w137) -> ("Rate Out"=w136:dbl)  [unwired: 2 in]
          }
          frame Enabled {
          }
        }
      }
    }
    n154 = feedback #5() -> (w113:T10)
    n155 = feedback-in #5(w113) -> ()
    n156 = case shown="True" w116 {
      tunnel: w115 -> [w209 w213]
      tunnel: w114 -> [w208 w212]
      tunnel: w113 -> [w210 w211]
      frame False {
        n157 = call <vilib>:"WPI_RobotDriveMotors.vi"("RightSpeed"=w208, "LeftSpeed"=w209, "RobotDriveDevRef"=w210) -> ()  [unwired: 6 in, 3 out]
      }
      frame True {
        n158 = call-poly <vilib>:"WPI_RobotDriveArcadeDrive.vi"("Y axis value"=w212, "X axis value"=w213, "RobotDriveDevRef"=w211) -> ()  [unwired: 6 in, 3 out]
      }
    }
    n159 = call "loop timer.vi"() -> ("IPS"=→"Main IPS":dbl, "SPI"=w126:u32)  [unwired: 1 in]
    "Main mSPI" <- w126
    n160 = call "performance fg.vi"("Menu"=fg_typedef."Get") -> ("Output"=w123:T9)  [unwired: 1 in]
    n161 = call "combined arm safety.vi"("Input"=w93) -> ("Safe Output"=w100:dbl, "Safety Data"=w95:T35)  [unwired: 13 in]
    n162 = call "dash safety data FG.vi"("Safety Data"=w95, "Menu"=fg_typedef."Set") -> ()  [unwired: 1 out]
    n163 = Bundle By Name(cluster=w123, "Main mSPI"=w126) -> (w122:T9)
    n164 = feedback #6() -> (w107:T11)
    n165 = feedback-in #6(w107) -> ()
    n166 = feedback #7() -> (w106:T11)
    n167 = feedback-in #7(w106) -> ()
    n168 = call <vilib>:"WPI_MotorControlSetOutput.vi"("Output"=w105, "MotorControlDevRef"=w107) -> ()  [unwired: 7 in, 3 out]
    n169 = call <vilib>:"WPI_MotorControlSetOutput.vi"("Output"=w100, "MotorControlDevRef"=w106) -> ()  [unwired: 7 in, 3 out]
    n170 = call "performance fg.vi"("Input"=w122, "Menu"=fg_typedef."Set") -> ()  [unwired: 1 out]
  }
  n171 = Merge Errors(w2, w1, "error in", w27, w26, w25, w24, w23, w22, w28) -> (→"error out":errorcluster)
